vi "Acquisition_5channels.vi"() -> ()   [LabVIEW 2014]
uses:
  <vilib>/eio/EIONode/EIONode.xnode
  <vilib>/rvi/DataTransferAndStorage/Container/XNode/niFpgaContainer.xnode
  <vilib>/rvi/eio/common/nirviEmuTemplateMethod_errors.vi
  <vilib>/rvi/interface/RandomDataEmulation/nirviRandomDataFpgaReadWriteTemplate.vi
  <vilib>/rvi/FIFO/Fifo_Resource/nirvififoEmulationRead.vi
  <vilib>/rvi/FIFO/Fifo_Resource/nirvififoEmulationWrite.vi
panel:
  out "Z-balanced 2":i16
  out "Z-balanced":bool
  out "Z-unbalanced":bool
  out "X":bool
  out "Y":bool
  out "X":i16
  out "Y":i16
  out "Z-unbalanced":i16
  out "Acquisition\nTimeout":bool
  in  "Sampling":u32 caption="Count(Ticks)"
  in  "DC-Sampling":u32 caption="Count(Ticks)"
  in  "Interleaving \nSampling":u32 caption="Count(Ticks)"
  in  "AOM-DC":i16
  in  "AOM update\nrate (ticks)":u32 caption="Count(Ticks)"
  out "AOM update":bool
  out "FIFO Z-unbalanced":bool
  out "FIFO Y":bool
  out "FIFO X":bool
  out "FIFO Z-balanced":bool
  out "data FIFO":bool
  out "FIFO-acquisition":bool
  out "DC component":i16
  out "DC FIFO":bool
  out "DC acquisition":bool
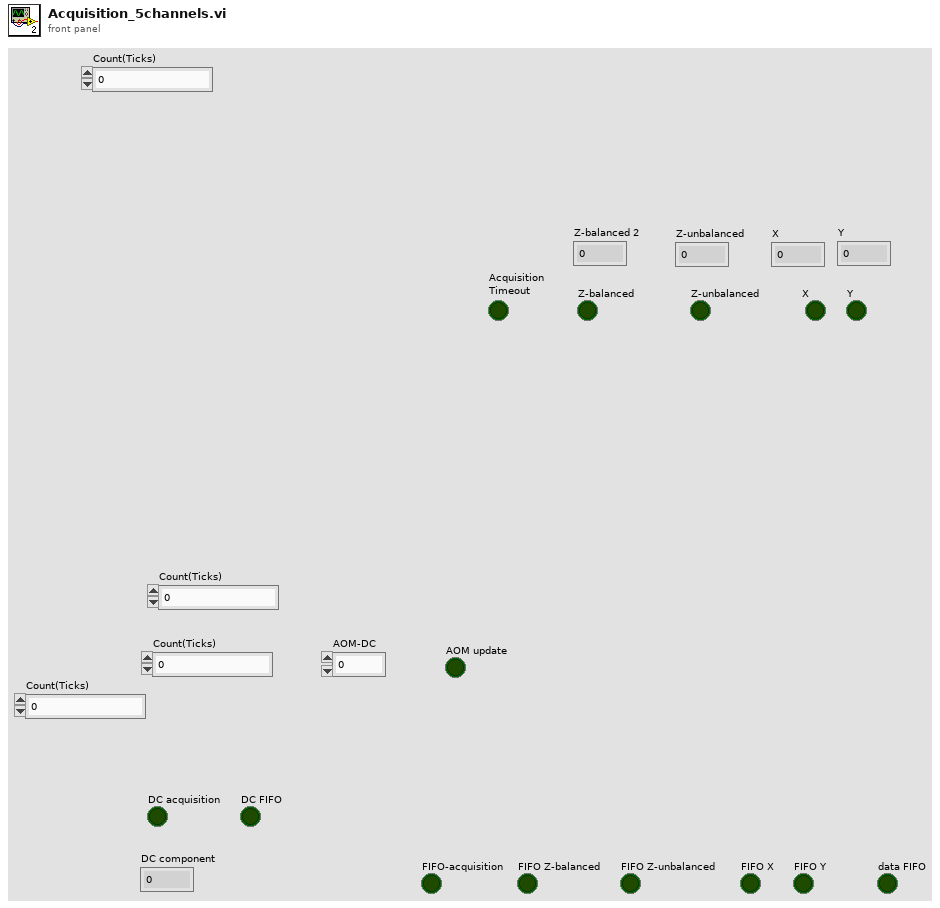
[diagram p1: front panel]
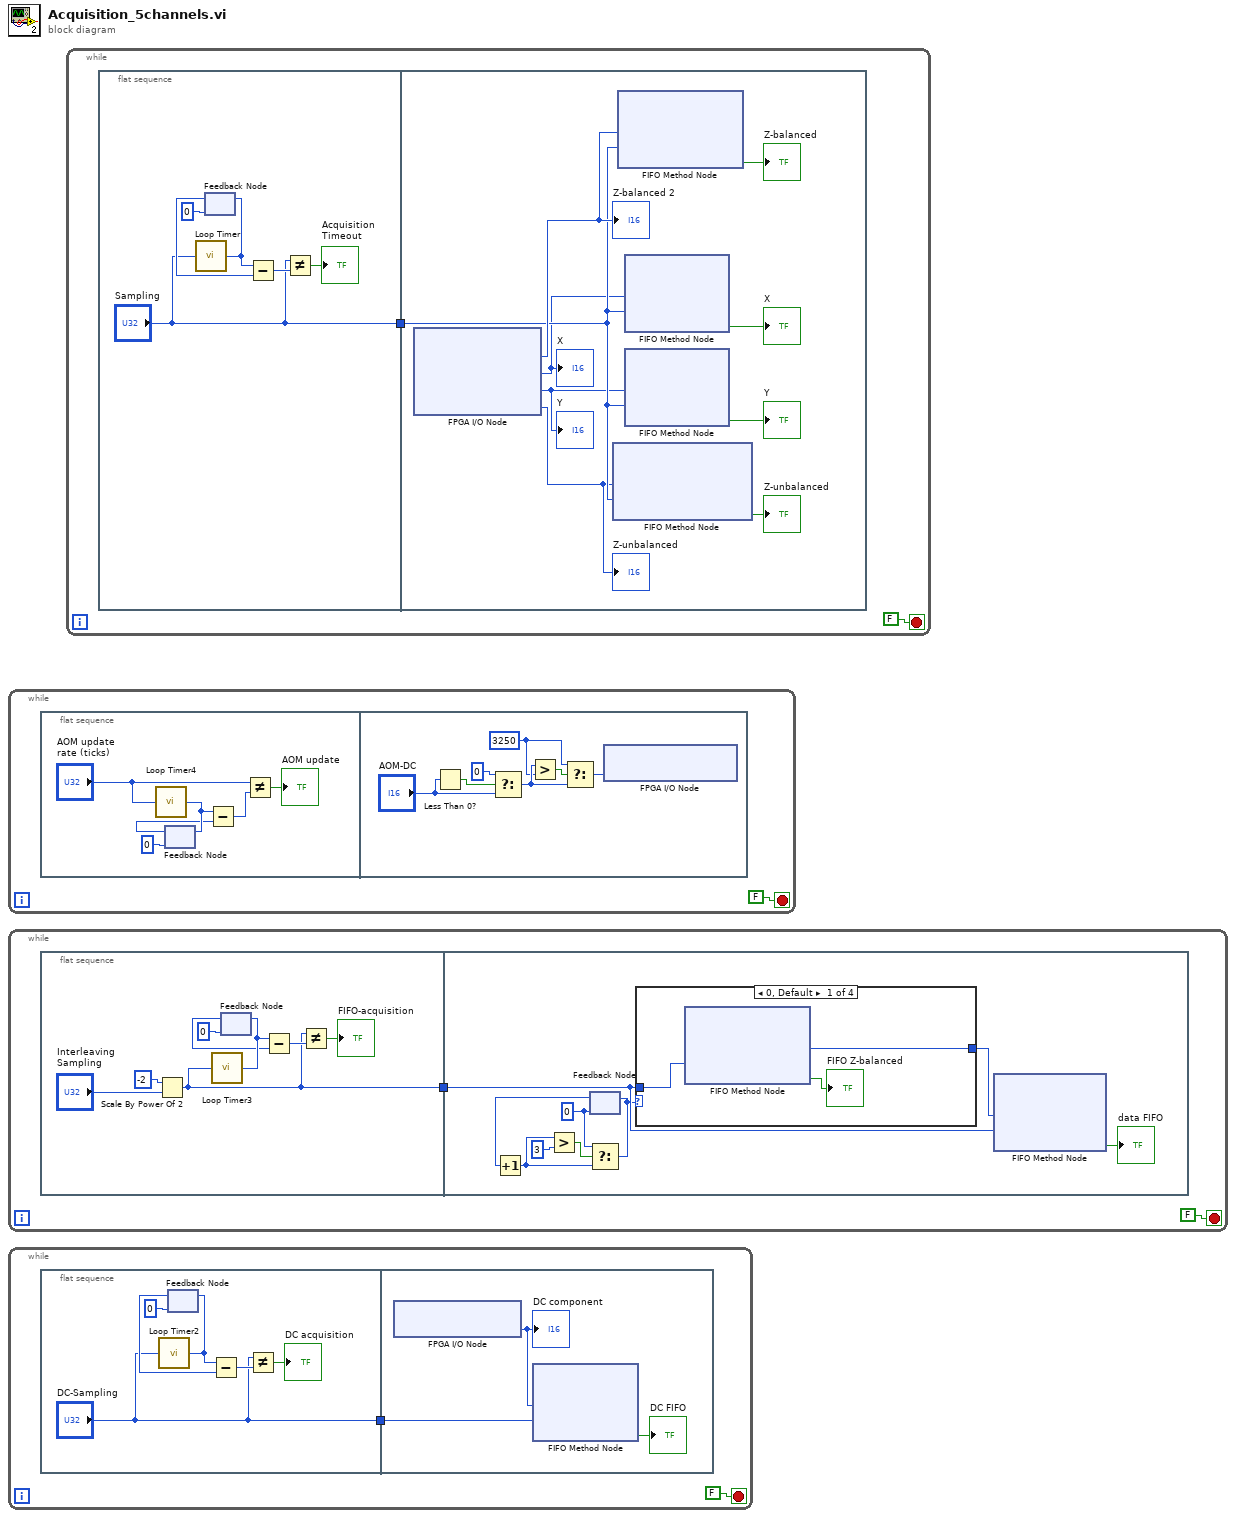
[diagram p0: block diagram]
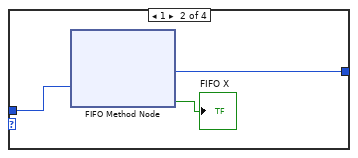
[diagram p2: hidden frame]
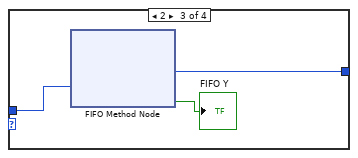
[diagram p3: hidden frame]
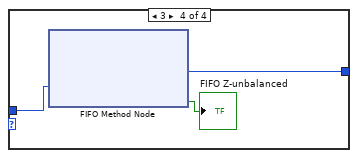
[diagram p4: hidden frame]
diagram:
  n1 = while {
    stop <- FALSE stop-if-true
    n2 = flat-sequence {
      frame #0 {
        n3 = call "Loop Timer4"("Count(Ticks)"="AOM update\nrate (ticks)") -> ("Tick Count(Ticks)"=w6:u32)
        n4 = feedback-in #1(w6) -> ()
        n5 = feedback #1(u32 0 ("Tick Count(Ticks)")) -> (w5:u32)
        n6 = Subtract(x=w6, y=w5) -> (x-y=w4:u32)
        n7 = Not Equal?(x="AOM update\nrate (ticks)", y=w4) -> (x != y?=→"AOM update":bool)
      }
      frame #1 {
        w8 = i16 3250
        n8 = Less Than 0?(x="AOM-DC") -> (x < 0?=w14:bool)
        n9 = Select(t=i16 0, s=w14, f="AOM-DC") -> (s? t:f=w11:i16)
        n10 = Greater?(x=w11, y=w8) -> (0:w12:bool)
        n11 = Select(t=w8, s=w12, f=w11) -> (s? t:f=w10:i16)
        n12 = xnode "FPGA I/O Node"("Connector0/AO5"=w10) -> ()  [unwired: 1 in, 1 out]
      }
    }
  }
  n13 = while {
    stop <- FALSE stop-if-true
    n14 = flat-sequence {
      tunnel: [w18] -> w15
      tunnel: w15 -> [w32]
      frame #0 {
        n15 = Scale By Power Of 2(n=i16 -2, x="Interleaving \nSampling") -> (x*2^n=w18:u32)
        n16 = call "Loop Timer3"("Count(Ticks)"=w18) -> ("Tick Count(Ticks)"=w23:u32)
        n17 = feedback-in #2(w23) -> ()
        n18 = feedback #2(u32 0 ("Tick Count(Ticks)")) -> (w22:u32)
        n19 = Subtract(x=w23, y=w22) -> (x-y=w21:u32)
        n20 = Not Equal?(x=w18, y=w21) -> (x != y?=→"FIFO-acquisition":bool)
      }
      frame #1 {
        w28 = i16 0
        n21 = feedback #3(w28) -> (w27:i16)
        n22 = Increment(x=w27) -> (x+1=w25:i16)
        n23 = Greater?(x=w25, y=i16 3) -> (0:w29:bool)
        n24 = Select(t=w28, s=w29, f=w25) -> (s? t:f=w26:i16)
        n25 = feedback-in #3(w26) -> ()
        n26 = case shown="0, Default" w26 {
          tunnel: w32 -> [w36 w37 w41 w43]
          tunnel: [w34 w39 w40 w44] -> w31
          frame 0, Default {
            n27 = xnode ("FIFO Method Node")("Timeout"=w36) -> ("Element"=w34:i16, "Timed Out?"=→"FIFO Z-balanced":bool)  [unwired: 1 in, 1 out]
          }
          frame 1 {
            n28 = xnode ("FIFO Method Node")("Timeout"=w37) -> ("Element"=w39:i16, "Timed Out?"=→"FIFO X":bool)  [unwired: 1 in, 1 out]
          }
          frame 2 {
            n29 = xnode ("FIFO Method Node")("Timeout"=w41) -> ("Element"=w40:i16, "Timed Out?"=→"FIFO Y":bool)  [unwired: 1 in, 1 out]
          }
          frame 3 {
            n30 = xnode ("FIFO Method Node")("Timeout"=w43) -> ("Element"=w44:i16, "Timed Out?"=→"FIFO Z-unbalanced":bool)  [unwired: 1 in, 1 out]
          }
        }
        n31 = xnode ("FIFO Method Node")("Element"=w31, "Timeout"=w32) -> ("Timed Out?"=→"data FIFO":bool)  [unwired: 1 in, 1 out]
      }
    }
  }
  n32 = while {
    stop <- FALSE stop-if-true
    n33 = flat-sequence {
      tunnel: ["DC-Sampling"] -> w46
      tunnel: w46 -> [w55]
      frame #0 {
        n34 = call "Loop Timer2"("Count(Ticks)"="DC-Sampling") -> ("Tick Count(Ticks)"=w52:u32)
        n35 = feedback-in #4(w52) -> ()
        n36 = feedback #4(u32 0 ("Tick Count(Ticks)")) -> (w51:u32)
        n37 = Subtract(x=w52, y=w51) -> (x-y=w50:u32)
        n38 = Not Equal?(x="DC-Sampling", y=w50) -> (x != y?=→"DC acquisition":bool)
      }
      frame #1 {
        n39 = xnode "FPGA I/O Node"() -> ("Connector0/AI7"=w56:i16)  [unwired: 1 in, 1 out]
        "DC component" <- w56
        n40 = xnode ("FIFO Method Node")("Element"=w56, "Timeout"=w55) -> ("Timed Out?"=→"DC FIFO":bool)  [unwired: 1 in, 1 out]
      }
    }
  }
  n41 = while {
    stop <- FALSE stop-if-true
    n42 = flat-sequence {
      tunnel: ["Sampling"] -> w57
      tunnel: w57 -> [w68]
      frame #0 {
        n43 = call "Loop Timer"("Count(Ticks)"="Sampling") -> ("Tick Count(Ticks)"=w63:u32)
        n44 = feedback-in #5(w63) -> ()
        n45 = feedback #5(u32 0 ("Tick Count(Ticks)")) -> (w62:u32)
        n46 = Subtract(x=w63, y=w62) -> (x-y=w61:u32)
        n47 = Not Equal?(x="Sampling", y=w61) -> (x != y?=→"Acquisition\nTimeout":bool)
      }
      frame #1 {
        n48 = xnode "FPGA I/O Node"() -> ("Connector0/AI6"=w72:i16, "Connector0/AI3"=w67:i16, "Connector0/AI4"=w66:i16, "Connector0/AI5"=w65:i16)  [unwired: 4 in, 4 out]
        "Z-balanced 2" <- w72
        "X" <- w67
        "Y" <- w66
        "Z-unbalanced" <- w65
        n49 = xnode ("FIFO Method Node")("Element"=w65, "Timeout"=w68) -> ("Timed Out?"=→"Z-unbalanced":bool)  [unwired: 1 in, 1 out]
        n50 = xnode ("FIFO Method Node")("Element"=w72, "Timeout"=w68) -> ("Timed Out?"=→"Z-balanced":bool)  [unwired: 1 in, 1 out]
        n51 = xnode ("FIFO Method Node")("Element"=w67, "Timeout"=w68) -> ("Timed Out?"=→"X":bool)  [unwired: 1 in, 1 out]
        n52 = xnode ("FIFO Method Node")("Element"=w66, "Timeout"=w68) -> ("Timed Out?"=→"Y":bool)  [unwired: 1 in, 1 out]
      }
    }
  }
